vi "BLSPowerSupplyTemplateService SetNumber.vi"(6 "contextId":T1, 8 "error in":errorcluster, 9 "timeout (ms)":i32=-1, 10 "Request Data":T3, 11 "gRPC ID":T1) -> (0 "error out":errorcluster, 2 "Response Data":T2, 3 "gRPC ID out":T1)   [LabVIEW 2023, in "BLSPowerSupplyTemplateService_client.lvlib"]
uses:
  BLSPowerSupplyTemplateService_client.lvlib
  <vilib>/gRPC/LabVIEW gRPC Library/Shared/grpcId.ctl
  RPC Messages/adas_SetNumberRequest.ctl
  RPC Messages/adas_Status.ctl
  14035477-4c25-4107-8ed5-d0c4ef420ce5.vi
  <vilib>/gRPC/LabVIEW gRPC Library/Shared/TranslateGrpcError.vi
  <vilib>/gRPC/LabVIEW gRPC Library/Shared/Wait On Occurence.vi
  <vilib>/gRPC/LabVIEW gRPC Library/Server API/Server/Get Server DLL Path.vi
  <vilib>/Utility/error.llb/Error Cluster From Error Code.vi
  <vilib>/gRPC/LabVIEW gRPC Library/grpc-lvsupport-release.lvlib
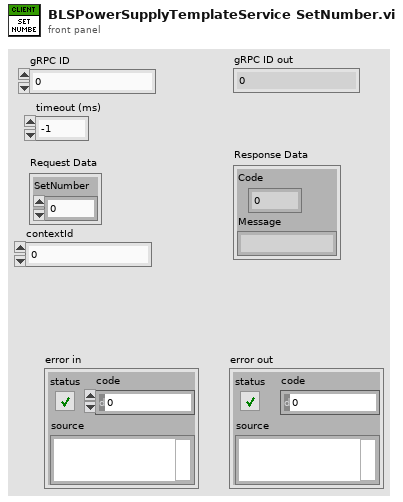
[diagram p1: front panel]
types:
  T1 = typedef "grpc-lvsupport-release.lvlib/grpcId.ctl" = u64
  T2 = typedef "BLSPowerSupplyTemplateService_client.lvlib/adas_Status.ctl" = cluster{"Code":i32, "Message":string}
  T3 = typedef "BLSPowerSupplyTemplateService_client.lvlib/adas_SetNumberRequest.ctl" = cluster{"SetNumber":u32}
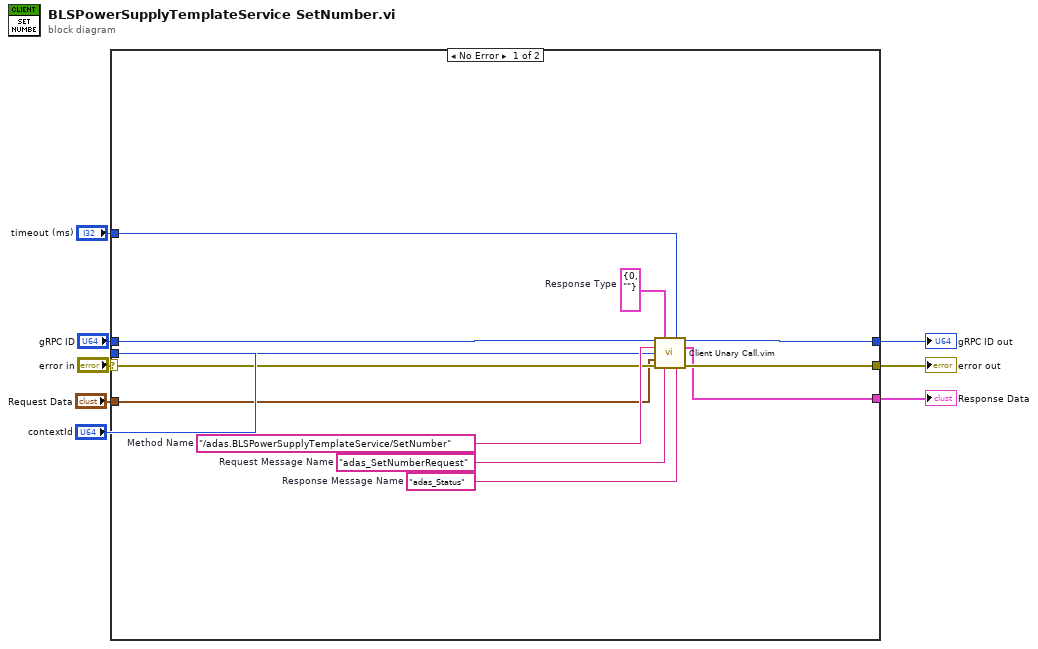
[diagram p0: block diagram]
diagram:
  n1 = case shown="No Error" "error in" {
    selector: "error in" -> [w16 w21]
    tunnel: [w15 w21] -> w7
    tunnel: "gRPC ID" -> [w14 w22]
    tunnel: [w13 w22] -> w5
    tunnel: "Request Data" -> [w12 _]
    tunnel: [w11 _] -> w3
    tunnel: "timeout (ms)" -> [w10 _]
    tunnel: "contextId" -> [w9 _]
    frame No Error {
      w17 = "adas_Status"  # Response Message Name
      w18 = "adas_SetNumberRequest"  # Request Message Name
      w19 = T2 {"Code"=0, "Message"=""}  # Response Type
      w20 = "/adas.BLSPowerSupplyTemplateService/SetNumber"  # Method Name
      n2 = call "Client Unary Call.vim"("ClientID in"=w14, "Response Type"=w19, "timeout (ms)"=w10, "Method Name"=w20, "contextId"=w9, "Request Data"=w12, "error in"=w16, "Request Message Name"=w18, "Response Message Name"=w17) -> ("ClientID out"=w13:u64, "Response Data"=w11:T2, "error out"=w15:errorcluster)  [unwired: 4 in]
    }
    frame Error {
    }
  }
  "error out" <- w7
  "gRPC ID out" <- w5
  "Response Data" <- w3
